vi "Connection_SET.vi"(8 "error in":errorcluster, 10 "connection":refnum<k5>, 11 "tcp server in":refnum<class "RT FlexRIO Server TCP.lvclass">) -> (0 "error out":errorcluster, 3 "tcp server out":refnum<class "RT FlexRIO Server TCP.lvclass">)   [LabVIEW 2017, in "RT FlexRIO Server TCP.lvclass"]
uses:
  RT FlexRIO Server TCP.lvclass
  RT FlexRIO Server TCP.lvclass/RT FlexRIO Server TCP.ctl
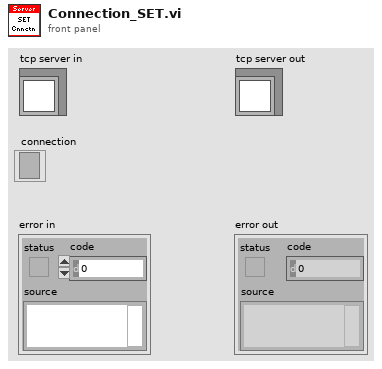
[diagram p1: front panel]
types:
  T1 = typedef "RT FlexRIO Server TCP.lvclass/SessionData.ctl" = cluster{"listener":refnum<k5>, "connection":refnum<k5>, "state":T2, "incoming":refnum<queue>, "outgoing":refnum<queue>, "state request":refnum<user-event>, "state changed":refnum<user-event>}
  T2 = typedef "RT FlexRIO Server TCP.lvclass/connection state.ctl" = enum16{"started", "connected", "stopped"}
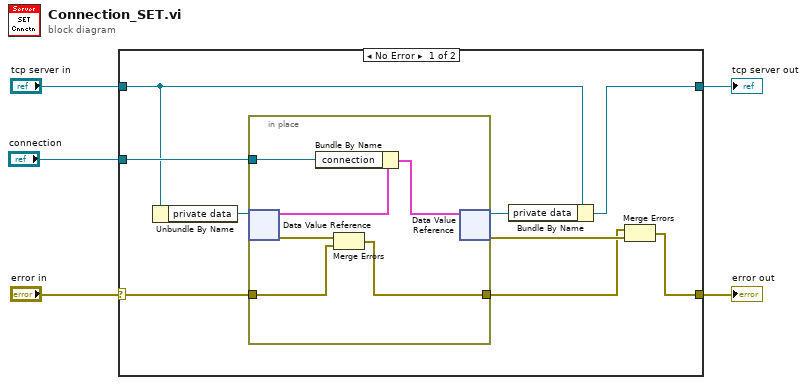
[diagram p0: block diagram]
diagram:
  n1 = case shown="No Error" "error in" {
    selector: "error in" -> [w13 w22]
    tunnel: [w10 w22] -> w4
    tunnel: "tcp server in" -> [w8 w21]
    tunnel: "connection" -> [w9 _]
    tunnel: [w6 w21] -> w2
    frame No Error {
      n2 = Unbundle By Name(w8) -> ("private data"=w14:refnum<data-value>)
      n3 = in-place {
        in-place-border: w13 -> [w19]
        in-place-border: [w18] -> w11
        in-place-border: w9 -> [w17]
        n4 = in-place-dvr #1(w14) -> (w16:T1, w20:errorcluster)
        n5 = Bundle By Name(cluster=w16, "connection"=w17) -> (w15:T1)
        n6 = Merge Errors(w20, w19) -> (w18:errorcluster)
        n7 = in-place-dvr #1(w15) -> (w7:refnum<data-value>, w12:errorcluster)
      }
      n8 = Bundle By Name(cluster=w8, "private data"=w7) -> (w6:refnum<class "RT FlexRIO Server TCP.lvclass">)
      n9 = Merge Errors(w11, w12) -> (w10:errorcluster)
    }
    frame Error {
    }
  }
  "error out" <- w4
  "tcp server out" <- w2
